vi "Get or Init BC Class Array.vi"(5 "type check? (T)":bool=TRUE, 7 "target BC":refnum<class "NI_BC.lvclass">, 8 "error in (no error)":errorcluster, 9 "index":i32, 10 "# of BC":i32, 11 "PDE in":refnum<class "NI_PDE.lvclass">) -> (0 "error out":errorcluster, 1 "BC out":refnum<class "NI_BC.lvclass">, 2 "BC Array":refnum<class "NI_BC.lvclass">[](array[class]), 3 "PDE out":refnum<class "NI_PDE.lvclass">)   [LabVIEW 2020, in "NI_PDE.lvlib" / "NI_PDE.lvclass"]
uses:
  <vilib>/gmath/pde.llb/PDEClass/NI_PDE.lvclass
  <vilib>/gmath/pde.llb/BCClass/NI_BC.lvclass
  <vilib>/gmath/pde.llb/BCClass/Class Type.ctl
  <vilib>/gmath/pde.llb/Common/PDE_Error.ctl
  <vilib>/gmath/NI_PDE.lvlib
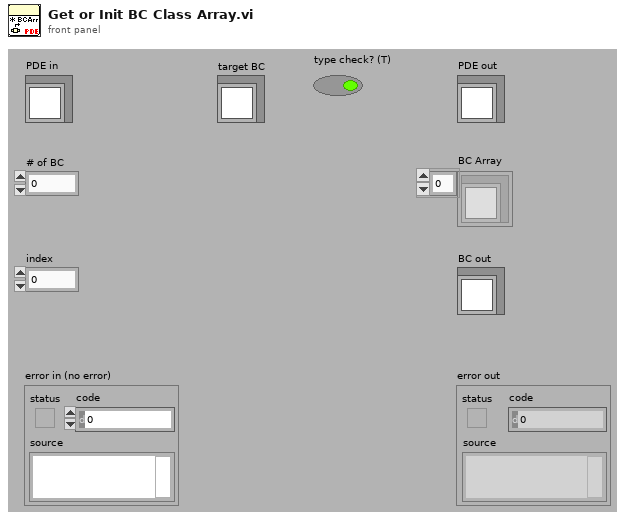
[diagram p1: front panel]
types:
  T1 = typedef "NI_PDE.lvlib/PDE_Error.ctl" = enum16{"No Error", "k is zero", "End point <= start point", "# of time steps < 2", "# of spatial points < 3", "# of grid < 1 for FEM", "# of boundary < 3 for FEM", "Incompatible RHS size", "Incompatible BC size", "Incompatible IC size", "PDE class conflict", "RHS class conflict", "Domain class conflict", "BC class conflict", "IC class conflict"}
  T2 = typedef "NI_PDE.lvlib/NI_BC.lvclass/Class Type.ctl" = i32
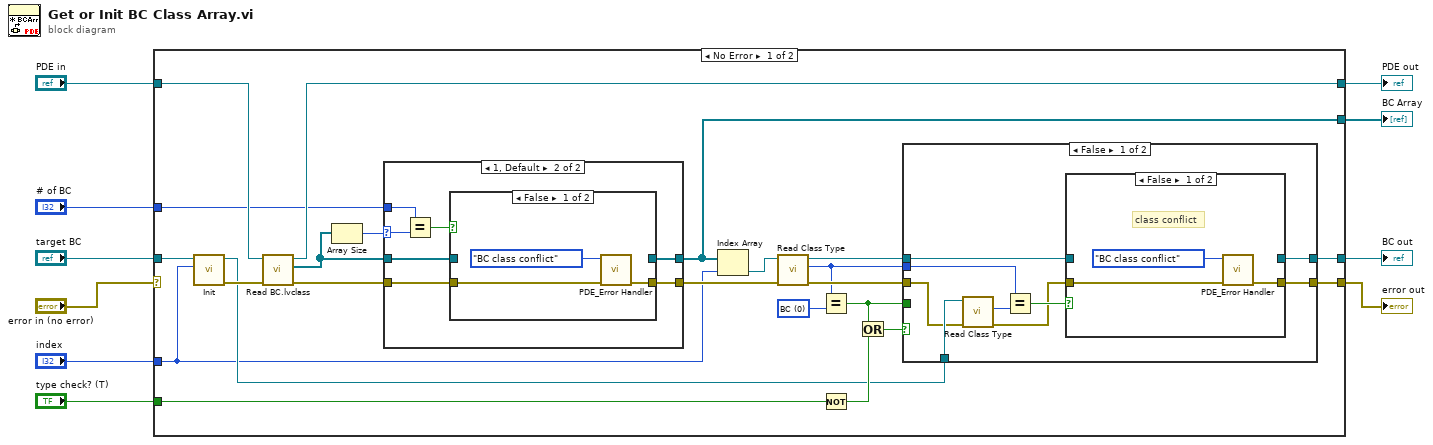
[diagram p0: block diagram]
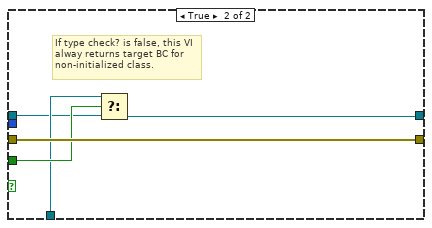
[diagram p3: hidden frame]
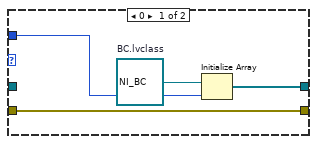
[diagram p4: hidden frame]
diagram:
  n1 = case shown="No Error" "error in (no error)" {
    selector: "error in (no error)" -> [_ w70]
    tunnel: "PDE in" -> [w33 w71]
    tunnel: [w24 w71] -> w9
    tunnel: [w23 w70] -> w8
    tunnel: "# of BC" -> [w22 _]
    tunnel: "index" -> [w11 _]
    tunnel: [w21 _] -> w5
    tunnel: [w20 w69] -> w4
    tunnel: "target BC" -> [w14 w69]
    tunnel: "type check? (T)" -> [w18 _]
    frame No Error {
      w28 = T2 0 items=["BC"=0, "BC_Steady"=100, "BC_Steady_2D"=120, "BC_Steady_2D_Numeric"=121, "BC_Steady_2D_VIRef"=122, "BC_Evolut"=200, "BC_Evolut_1D"=210, "BC_Evolut_1D_Numeric"=211, "BC_Evolut_1D_VIRef"=212, "BC_Evolut_2D"=220, "BC_Evolut_2D_Numeric"=221, "BC_Evolut_2D_VIRef"=222] ("y")
      n2 = call-dynamic "Init.vi"("index"=w11, "BC"=w14) -> ("error out"=w13:errorcluster, "initialized BC"=w12:refnum<class "NI_BC.lvclass">)  [unwired: 1 in, 7 out]
      n3 = call-dynamic "Read BC.lvclass.vi"("error in (no error)"=w13, "PDE.lvclass in"=w33) -> ("error out"=w31:errorcluster, "BC.lvclass"=w30:refnum<class "NI_BC.lvclass">[], "PDE.lvclass out"=w24:refnum<class "NI_PDE.lvclass">)  [unwired: 7 out]
      n4 = Array Size(array=w30) -> (size(s)=w32:i32)
      n5 = case shown="1, Default" w32 {
        selector: w32 -> [_ w60]
        tunnel: w31 -> [w55 w63]
        tunnel: [w54 w57] -> w21
        tunnel: w30 -> [_ w58]
        tunnel: [w55 w62] -> w25
        tunnel: w22 -> [w53 w61]
        frame 0 {
          w56 = refnum<class "NI_BC.lvclass"> refnum  # BC.lvclass
          n6 = Initialize Array(w56, w53) -> (w54:refnum<class "NI_BC.lvclass">[])
        }
        frame 1, Default {
          n7 = Equal?(x=w61, y=w60) -> (x = y?=w59:bool)
          n8 = case shown="False" w59 {
            tunnel: w63 -> [w65 w67]
            tunnel: [w64 w67] -> w62
            tunnel: w58 -> [_ w68]
            tunnel: [_ w68] -> w57
            frame False {
              n9 = call <vilib>:"PDE_Error Handler.vi"("error in (no error)"=w65, "PDE error"=PDE_Error."BC class conflict") -> ("error out"=w64:errorcluster)  [unwired: 9 out]
            }
            frame True {
            }
          }
        }
      }
      n10 = Index Array(array=w21, index=w11) -> (element=w29:refnum<class "NI_BC.lvclass">)
      n11 = call-dynamic "Read Class Type.vi"("error in (no error)"=w25, "BC.lvclass in"=w29) -> ("error out"=w26:errorcluster, "BC class type"=w19:T2, "BC.lvclass out"=w27:refnum<class "NI_BC.lvclass">)  [unwired: 7 out]
      n12 = Equal?(x=w19, y=w28) -> (x = y?=w15:bool)
      n13 = Not(x=w18) -> (.not. x?=w17:bool)
      n14 = Or(x=w15, y=w17) -> (x .or. y?=w16:bool)
      n15 = case shown="False" w16 {
        tunnel: w27 -> [w42 w49]
        tunnel: w26 -> [w35 w52]
        tunnel: [w41 w52] -> w23
        tunnel: [w40 w48] -> w20
        tunnel: w19 -> [w39 _]
        tunnel: w12 -> [w37 w50]
        tunnel: w15 -> [_ w51]
        frame False {
          n16 = call-dynamic "Read Class Type.vi"("error in (no error)"=w35, "BC.lvclass in"=w37) -> ("error out"=w34:errorcluster, "BC class type"=w36:T2)  [unwired: 8 out]
          n17 = Equal?(x=w39, y=w36) -> (x = y?=w38:bool)
          n18 = case shown="False" w38 {
            tunnel: w42 -> [_ w47]
            tunnel: w34 -> [w44 w46]
            tunnel: [_ w47] -> w40
            tunnel: [w43 w46] -> w41
            frame False {
              # "class conflict"
              n19 = call <vilib>:"PDE_Error Handler.vi"("error in (no error)"=w44, "PDE error"=PDE_Error."BC class conflict") -> ("error out"=w43:errorcluster)  [unwired: 9 out]
            }
            frame True {
            }
          }
        }
        frame True {
          # "If type check? is false, this VI alway returns target BC for non-initialized class."
          n20 = Select(t=w50, s=w51, f=w49) -> (s? t:f=w48:refnum<class "NI_BC.lvclass">)
        }
      }
    }
    frame Error {
    }
  }
  "PDE out" <- w9
  "error out" <- w8
  "BC Array" <- w5
  "BC out" <- w4
